vi "Load and Save Data (List-formatted Data).vi"(0 "VISA resource name":refnum<visa-resource-name>, 5 "Destination File":string, 7 "8-bit Values":u32[](array[numeric])=[0], 11 "error in (no error)":errorcluster) -> (4 "VISA resource name out":refnum<visa-resource-name>, 15 "error out":errorcluster)   [LabVIEW 2018, in "Agilent PSG MXG Series.lvlib"]
doc: "Loads list-formatted data directly into pattern RAM volatile memory (WFM1). Pattern RAM memory describes how memory (WFM1) is used and is not a distinct piece of memory. A PRAM file is specified as an array of bytes.\n\n<B>Note:</B>\nThis VI is only valid in N5172B that installs with <B>Option 653</B> or <B>Option 655</B>, or N5182B that installs with <B>Option 656</B> or <B>Option 657</B>."
uses:
  Agilent PSG MXG Series.lvlib
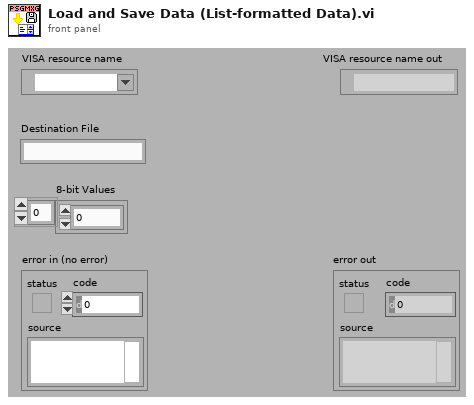
[diagram p1: front panel]
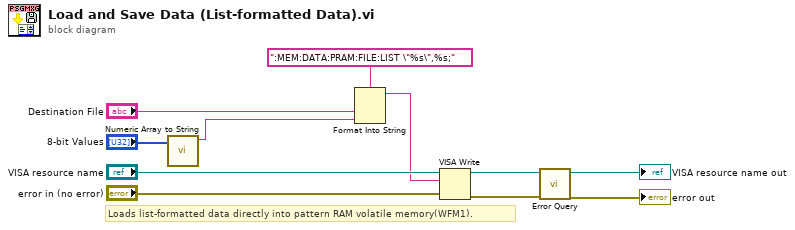
[diagram p0: block diagram]
diagram:
  # "Loads list-formatted data directly into pattern RAM volatile memory(WFM1)."
  n1 = call "Numeric Array to String.vi"("Numeric Array"="8-bit Values") -> ("Output String"=w1:string)  [unwired: 10 in]
  n2 = Format Into String(format string=":MEM:DATA:PRAM:FILE:LIST \"%s\",%s;", "Destination File", w1) -> (resulting string=w4:string)  [unwired: 2 in, 1 out]
  n3 = VISA Write(VISA resource name="VISA resource name", write buffer=w4, error in (no error)="error in (no error)") -> (VISA resource name out=w11:refnum<visa-resource-name>, error out=w10:errorcluster)  [unwired: 1 out]
  n4 = call "Error Query.vi"("error in (no error)"=w10, "VISA resource name"=w11) -> ("error out"=→"error out":errorcluster, "VISA resource name out"=→"VISA resource name out":refnum<visa-resource-name>)  [unwired: 6 in, 2 out]
